vi "Release message Queues.vi"(8 "error in":errorcluster, 11 "Messages":T1) -> (0 "error out":errorcluster)   [LabVIEW 2019, in "Messages.lvlib"]
doc: "This VI creates and initializes all the message queues for your application. If your application requires more than one message queue, right-click the \"Message Queues\" constant above and select Open Type Def. Add the new Message Queue(s) to the type definition, then initialize them in this VI."
uses:
  Messages.lvlib
  ctl/Messages.ctl
  <vilib>/NI/AMC/Message Queue.ctl
  <vilib>/NI/AMC/Message.ctl
  <vilib>/NI/Tools/Keyed Array/KeyedArray.ctl
  <vilib>/NI/Tools/Keyed Array/Tools_KeyedArray.lvlib
  <vilib>/NI/AMC/AMC.lvlib
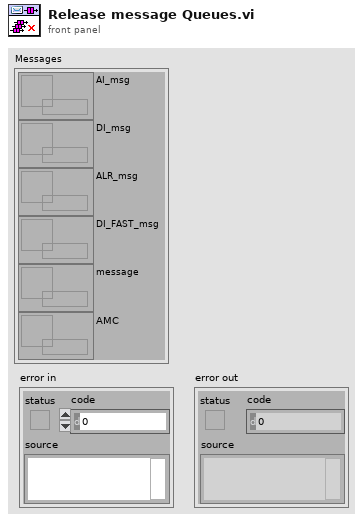
[diagram p1: front panel]
types:
  T1 = typedef "Messages.lvlib/Messages.ctl" = cluster{"AI_msg":refnum<queue>, "DI_msg":refnum<queue>, "ALR_msg":refnum<queue>, "DI_FAST_msg":refnum<queue>, "message":refnum<queue>, "AMC":T2}
  T2 = typedef "AMC.lvlib/Message Queue.ctl" = refnum<queue>
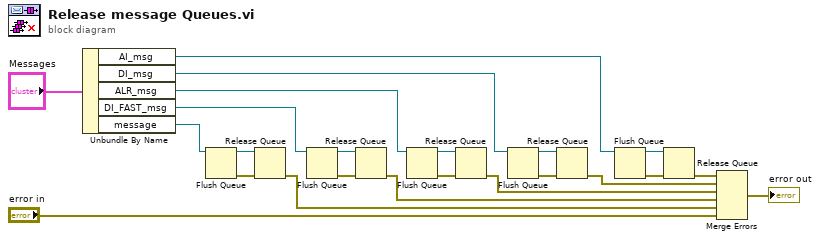
[diagram p0: block diagram]
diagram:
  n1 = Unbundle By Name("Messages") -> ("AI_msg"=w9:refnum<queue>, "DI_msg"=w11:refnum<queue>, "ALR_msg"=w12:refnum<queue>, "DI_FAST_msg"=w17:refnum<queue>, "message"=w20:refnum<queue>)
  n2 = Flush Queue(queue=w20) -> (queue out=w22:refnum<queue>, error out=w21:errorcluster)  [unwired: 1 in, 1 out]
  n3 = Release Queue(queue=w22, error in (no error)=w21) -> (error out=w4:errorcluster)  [unwired: 1 in, 2 out]
  n4 = Flush Queue(queue=w17) -> (queue out=w18:refnum<queue>, error out=w19:errorcluster)  [unwired: 1 in, 1 out]
  n5 = Release Queue(queue=w18, error in (no error)=w19) -> (error out=w5:errorcluster)  [unwired: 1 in, 2 out]
  n6 = Flush Queue(queue=w12) -> (queue out=w13:refnum<queue>, error out=w14:errorcluster)  [unwired: 1 in, 1 out]
  n7 = Release Queue(queue=w13, error in (no error)=w14) -> (error out=w6:errorcluster)  [unwired: 1 in, 2 out]
  n8 = Flush Queue(queue=w11) -> (queue out=w16:refnum<queue>, error out=w15:errorcluster)  [unwired: 1 in, 1 out]
  n9 = Release Queue(queue=w16, error in (no error)=w15) -> (error out=w7:errorcluster)  [unwired: 1 in, 2 out]
  n10 = Flush Queue(queue=w9) -> (queue out=w1:refnum<queue>, error out=w10:errorcluster)  [unwired: 1 in, 1 out]
  n11 = Release Queue(queue=w1, error in (no error)=w10) -> (error out=w8:errorcluster)  [unwired: 1 in, 2 out]
  n12 = Merge Errors(w8, w7, w6, w5, w4, "error in") -> (→"error out":errorcluster)
